vi "In Range.vi"(9 "lower limit":dbl, 10 "upper limit":dbl, 11 "x":dbl) -> (3 "f":i8)   [LabVIEW 2016]
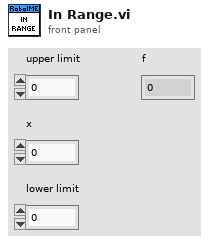
[diagram p1: front panel]
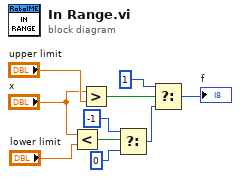
[diagram p0: block diagram]
diagram:
  n1 = Less?(x="x", y="lower limit") -> (x < y?=w6:bool)
  n2 = Greater?(x="x", y="upper limit") -> (0:w2:bool)
  n3 = Select(t=i8 -1, s=w6, f=i8 0) -> (s? t:f=w9:i8)
  n4 = Select(t=i8 1, s=w2, f=w9) -> (s? t:f=→"f":i8)
